vi "Get List Index.vi"(8 "error in (no error)":errorcluster, 9 "displayed errors":T1[](array[typedef]), 10 "coords":T2, 11 "error list":refnum<vi>) -> (0 "error out":errorcluster, 3 "index":T1)   [LabVIEW 2017]
uses:
  Error List/Error Owner and ID.ctl
  <vilib>/Utility/miscctls.llb/LVPoint32TypeDef.ctl
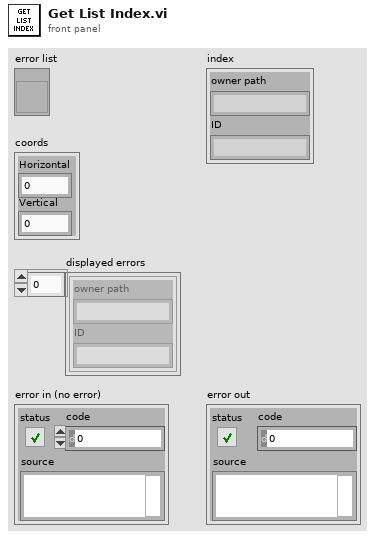
[diagram p1: front panel]
types:
  T1 = typedef "Error Owner and ID.ctl" = cluster{"owner path":string, "ID":string}
  T2 = typedef "LVPoint32TypeDef.ctl" = cluster{"Horizontal":i32, "Vertical":i32}
  T3 = typedef "LVRowAndColumnTypeDef.ctl" = cluster{"Row":i32, "Column":i32}
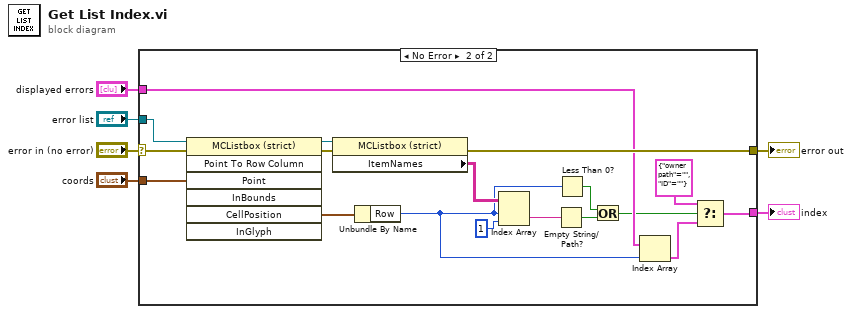
[diagram p0: block diagram]
diagram:
  n1 = case shown="No Error" "error in (no error)" {
    selector: "error in (no error)" -> [w7 w17]
    tunnel: [_ w15] -> w6
    tunnel: "coords" -> [_ w21]
    tunnel: "error list" -> [_ w20]
    tunnel: [w7 w18] -> w2
    tunnel: "displayed errors" -> [_ w13]
    frame Error {
    }
    frame No Error {
      n2 = invoke class="MCListbox (strict)" method="Point To Row Column"(reference=w20, error in=w17, "Point"=w21) -> (reference out=w23:refnum<vi>, error out=w19:errorcluster, "CellPosition"=w22:T3)  [unwired: 4 in, 4 out]
      n3 = property class="MCListbox (strict)"(reference=w23, error in=w19) -> (error out=w18:errorcluster, "ItemNames"=w24:string[][])  [unwired: 1 out]
      n4 = Unbundle By Name(w22) -> ("Row"=w8:i32)
      n5 = Index Array(array=w24, index (row)=w8, index (col)=1 ("disabled index (col)")) -> (element=w16:string)
      n6 = Empty String/Path?(string/path=w16) -> (empty?=w11:bool)
      n7 = Less Than 0?(x=w8) -> (x < 0?=w9:bool)
      n8 = Or(x=w9, y=w11) -> (x .or. y?=w10:bool)
      n9 = Index Array(array=w13, index=w8) -> (element=w14:T1)
      n10 = Select(t=T1 {"owner path"="", "ID"=""}, s=w10, f=w14) -> (s? t:f=w15:T1)
    }
  }
  "index" <- w6
  "error out" <- w2
